vi "Supports Terminal.vi"(8 "error in (no error)":errorcluster, 11 "Resource in":refnum<class "Resource.lvclass">) -> (0 "error out":errorcluster, 2 "Supports Terminal":bool, 3 "Resource out":refnum<class "Resource.lvclass">)   [LabVIEW 2020, in "PicoG-Core.lvlib" / "Resource.lvclass"]
doc: "This property determines whether the resource supports the IG Stream Terminal functionality or not. This should generally be true for Resource implementations that wrap an IG Stream implementation and false otherwise. To provide support, a child class must override this property to return a true value and also override the Connection property to supply the stream that can be utilized with the terminal."
uses:
  Resource.lvclass
  Resource.lvclass/Resource.ctl
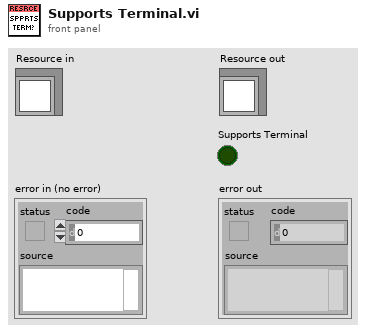
[diagram p1: front panel]
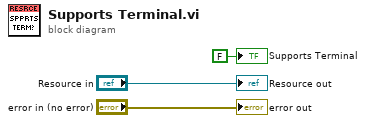
[diagram p0: block diagram]
diagram:
  "error out" <- "error in (no error)"
  "Resource out" <- "Resource in"
  "Supports Terminal" <- FALSE ("Supports Terminal")
